vi "inst parameters to array.vi"(11 "Input":T1 {"Array" format="%#_6p"}) -> (3 "Array":dbl[](array[numeric]))   [LabVIEW 2020, in "Measurement.lvclass"]
uses:
  Measurement.lvclass
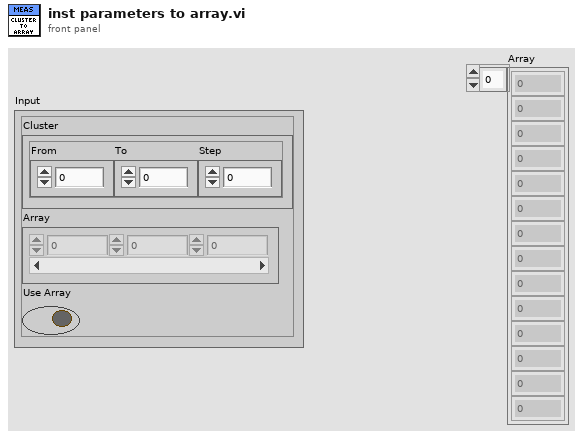
[diagram p1: front panel]
types:
  T1 = cluster{"Cluster ":cluster{"From":dbl, "To":dbl, "Step":dbl}, "Array":dbl[], "Use Array":bool}
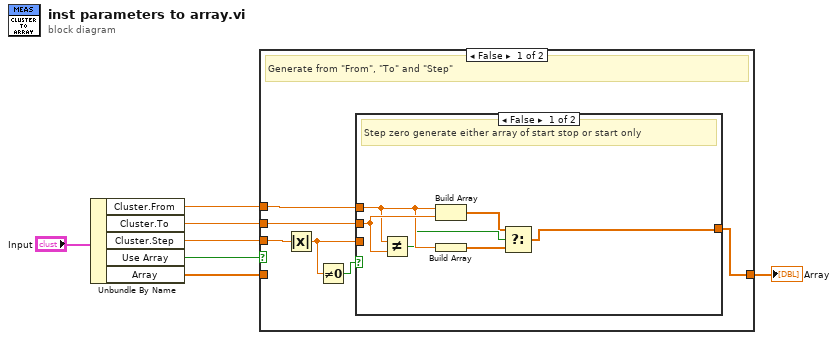
[diagram p0: block diagram]
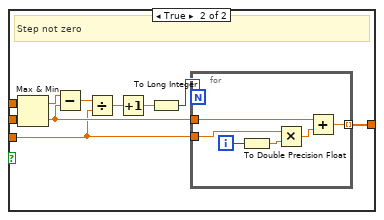
[diagram p2: hidden frame]
diagram:
  n1 = Unbundle By Name("Input") -> ("Cluster.From"=w5:dbl, "Cluster.To"=w4:dbl, "Cluster.Step"=w3:dbl, "Use Array"=w7:bool, "Array"=w6:dbl[])
  n2 = case shown="False" w7 {
    tunnel: w6 -> [_ w36]
    tunnel: [w10 w36] -> w2
    tunnel: w5 -> [w13 _]
    tunnel: w4 -> [w12 _]
    tunnel: w3 -> [w11 _]
    frame False {
      # "Generate from \"From\", \"To\" and \"Step\""
      n3 = Absolute Value(x=w11) -> (abs(x)=w8:dbl)
      n4 = Not Equal To 0?(x=w8) -> (x != 0?=w9:bool)
      n5 = case shown="False" w9 {
        tunnel: w13 -> [w18 w29]
        tunnel: w12 -> [w19 w28]
        tunnel: [w14 w21] -> w10
        tunnel: w8 -> [_ w20]
        frame False {
          # "Step zero generate either array of start stop or start only"
          n6 = Not Equal?(x=w18, y=w19) -> (x != y?=w17:bool)
          n7 = Build Array(w18, w19) -> (w15:dbl[])
          n8 = Build Array(w18) -> (w16:dbl[])
          n9 = Select(t=w15, s=w17, f=w16) -> (s? t:f=w14:dbl[])
        }
        frame True {
          # "Step not zero"
          n10 = Max & Min(x=w29, y=w28) -> (max(x,y)=w27:dbl, min(x,y)=w22:dbl)
          n11 = Subtract(x=w27, y=w22) -> (x-y=w26:dbl)
          n12 = Divide(x=w26, y=w20) -> (x/y=w25:dbl)
          n13 = Increment(x=w25) -> (x+1=w24:dbl)
          n14 = To Long Integer(number=w24) -> (32bit integer=w23:i32)
          n15 = for {
            N: w23 -> [_]
            tunnel: w22 -> [w31]
            tunnel: w20 -> [w34]
            tunnel: [w30] -> w21 mode=indexing
            i -> [w35]
            n16 = To Double Precision Float(number=w35) -> (double precision float=w33:dbl)
            n17 = Multiply(x=w34, y=w33) -> (x*y=w32:dbl)
            n18 = Add(x=w31, y=w32) -> (x+y=w30:dbl)
          }
        }
      }
    }
    frame True {
      # "Use the Array"
    }
  }
  "Array" <- w2
